vi "Cluster.vi"() -> ()   [LabVIEW 2015]
panel:
  out "Cluster Indicator":T1 {"Temp" scale=0.0..200.0; "Level" scale=0.0..10.0}
  in  "Password":string
  in  "Cluster":T1 {"Temp" scale=0.0..200.0; "Level" scale=0.0..10.0}
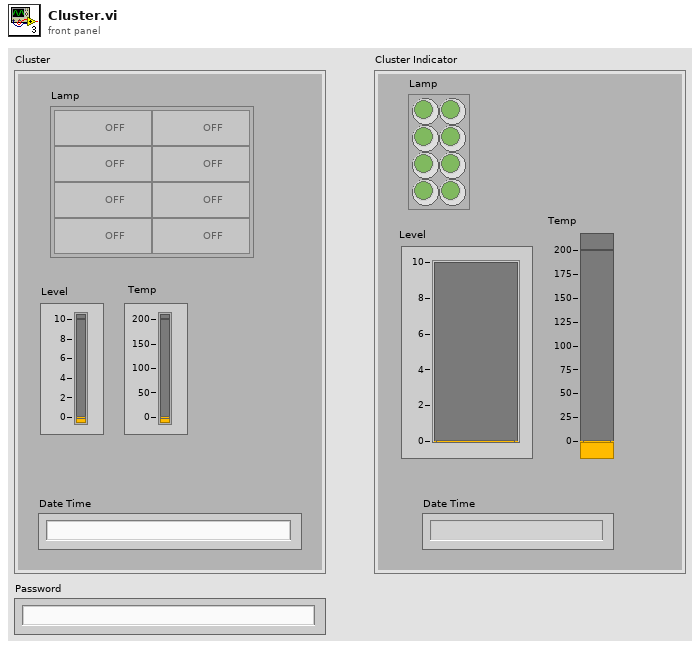
[diagram p1: front panel]
types:
  T1 = cluster{"Lamp":bool[][], "Level":dbl, " Temp":dbl, "Date Time ":string}
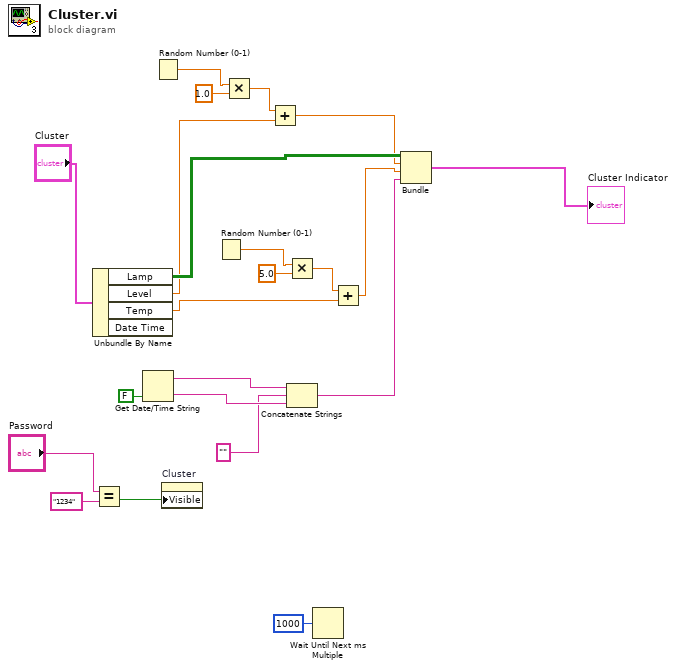
[diagram p0: block diagram]
diagram:
  n1 = Unbundle By Name "Unbundle By Name"("Cluster") -> ("Lamp"=w20:bool[][], "Level"=w11:dbl, "Temp"=w4:dbl)  [unwired: 1 out]
  n2 = Equal?(x="Password", y="1234") -> (x = y?=w1:bool)
  n3 = Get Date/Time String(want seconds? (F)=FALSE) -> (date string=w19:string, time string=w18:string)  [unwired: 2 in]
  n4 = Random Number (0-1)() -> (number: 0 to 1=w9:dbl)
  n5 = property on="Cluster" class="Clust (strict)"("Visible"=w1) -> ()  [unwired: 2 in, 2 out]
  n6 = Random Number (0-1)() -> (number: 0 to 1=w6:dbl)
  n7 = Multiply(x=w9, y=1.0) -> (x*y=w12:dbl)
  n8 = Add(x=w12, y=w11) -> (x+y=w10:dbl)
  n9 = Multiply(x=w6, y=5.0) -> (x*y=w5:dbl)
  n10 = Concatenate Strings "Concatenate Strings"(w19, "" ("string"), w18) -> (w17:string)
  n11 = Wait Until Next ms Multiple(millisecond multiple=u32 1000) -> ()  [unwired: 1 out]
  n12 = Add(x=w5, y=w4) -> (x+y=w3:dbl)
  n13 = Bundle "Bundle"("Lamp"=w20, w10, w3, w17) -> (→"Cluster Indicator":cluster{"Lamp":bool[][], dbl, dbl, string})  [unwired: 1 in]
